vi "Read SP LOCAL Comm Parameters.vi"(8 "error in (no error)":errorcluster, 11 "SemiProbe in":refnum<class "SemiProbe.lvclass">) -> (0 "error out":errorcluster, 2 "SP LOCAL Comm Parameters":T1={"address"="localhost", "port"=5050, "SP TCP Cnx ID"=refnum, "mode (standard)"=enum."Immediate", "bytes to read"=300, "timeout (ms)"=1000000}, 3 "SemiProbe out":refnum<class "SemiProbe.lvclass">)   [LabVIEW 2018, in "SemiProbe.lvclass"]
uses:
  SemiProbe.lvclass
  SemiProbe.lvclass/SemiProbe.ctl
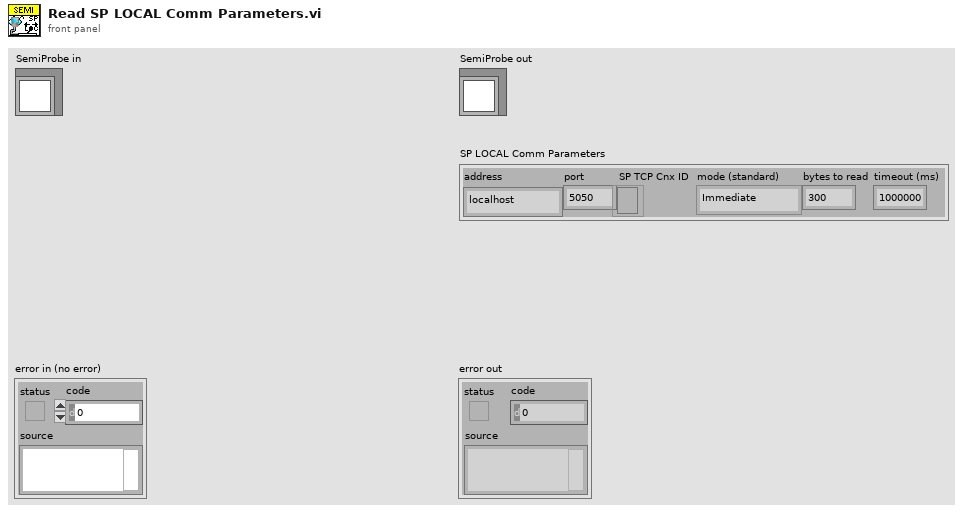
[diagram p1: front panel]
types:
  T1 = cluster{"address":string, "port":i32, "SP TCP Cnx ID":refnum<k5>, "mode (standard)":enum16{"Standard", "Buffered", "CRLF", "Immediate"}, "bytes to read":i32, "timeout (ms)":i32}
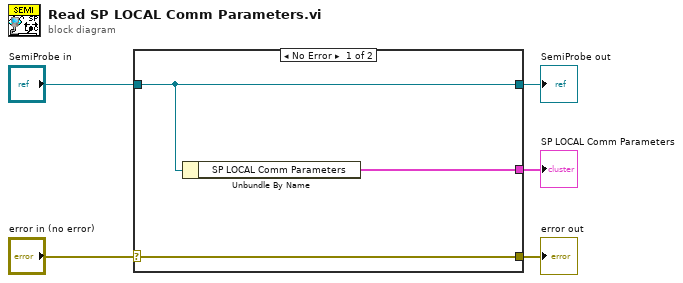
[diagram p0: block diagram]
diagram:
  n1 = case shown="No Error" "error in (no error)" {
    selector: "error in (no error)" -> [w8 w9]
    tunnel: [w8 w9] -> w4
    tunnel: [w7 w10] -> w2
    tunnel: "SemiProbe in" -> [w7 w10]
    tunnel: [w6 _] -> w1
    frame No Error {
      n2 = Unbundle By Name(w7) -> ("SP LOCAL Comm Parameters"=w6:T1)
    }
    frame Error {
    }
  }
  "error out" <- w4
  "SemiProbe out" <- w2
  "SP LOCAL Comm Parameters" <- w1
